vi "rsidr_core_global.vi"() -> ()   [LabVIEW 2015, in "Rohde&Schwarz CMXP GPRF.lvlib"] (continued)
i0, i1, i2, i3, i4, i5, i6, i7, i8, i9, i10, i11, i12, i13, i14, i15, i16, i17, i18, i19, i20, i21, i22, i23, i24, i25, i26, i27, i28, i29, i30, i31, i32\r\n\nRemote-control command(s):\nREAD:GPRF:MEAS<i>:IQRecorder:BIN?"}, {"Level"=3, "Class Only"=FALSE, "Identifier"="RSCMXPGPRF_ATTR_READ_IQ_RECORDER_MEASUREMENT_IQ_AMPLITUDES", "Descriptive Name"="Read IQ Recorder Measurement IQ Amplitudes", "Data Type"=6, "Command"="READ:GPRF:MEAS{instance}:IQR?", "Access"=0, "Range Table"="", "Read Callback"="", "Write Callback"="", "Supported Models"="", "Instrument Options"="", "Flags"=0, "Help"="Returns the I and Q amplitudes in the format specified by FORMat:BASE:DATA.\n\nAvailable Repeated Capabilities:\ninstance: i0, i1, i2, i3, i4, i5, i6, i7, i8, i9, i10, i11, i12, i13, i14, i15, i16, i17, i18, i19, i20, i21, i22, i23, i24, i25, i26, i27, i28, i29, i30, i31, i32\r\n\nRemote-control command(s):\nREAD:GPRF:MEAS<i>:IQRecorder?"}, {"Level"=3, "Class Only"=FALSE, "Identifier"="RSCMXPGPRF_ATTR_FETCH_IQ_RECORDER_MEASUREMENT_IQ_AMPLITUDES", "Descriptive Name"="Fetch IQ Recorder Measurement IQ Amplitudes", "Data Type"=6, "Command"="FETC:GPRF:MEAS{instance}:IQR?", "Access"=0, "Range Table"="", "Read Callback"="", "Write Callback"="", "Supported Models"="", "Instrument Options"="", "Flags"=0, "Help"="Returns the I and Q amplitudes in the format specified by FORMat:BASE:DATA.\n\nAvailable Repeated Capabilities:\ninstance: i0, i1, i2, i3, i4, i5, i6, i7, i8, i9, i10, i11, i12, i13, i14, i15, i16, i17, i18, i19, i20, i21, i22, i23, i24, i25, i26, i27, i28, i29, i30, i31, i32\r\n\nRemote-control command(s):\nFETCh:GPRF:MEAS<i>:IQRecorder?"}, {"Level"=3, "Class Only"=FALSE, "Identifier"="RSCMXPGPRF_ATTR_FETCH_IQ_RECORDER_MEASUREMENT_RELIABILITY", "Descriptive Name"="Fetch IQ Recorder Measurement Reliability", "Data Type"=6, "Command"="FETC:GPRF:MEAS{instance}:IQR:REL?", "Access"=0, "Range Table"="", "Read Callback"="", "Write Callback"="", "Supported Models"="", "Instrument Options"="", "Flags"=0, "Help"="Queries the reliability indicator for the I/Q recorder, see Reliability Indicator.\n\nAvailable Repeated Capabilities:\ninstance: i0, i1, i2, i3, i4, i5, i6, i7, i8, i9, i10, i11, i12, i13, i14, i15, i16, i17, i18, i19, i20, i21, i22, i23, i24, i25, i26, i27, i28, i29, i30, i31, i32\r\n\nRemote-control command(s):\nFETCh:GPRF:MEAS<i>:IQRecorder:RELiability?"}, {"Level"=1, "Class Only"=TRUE, "Identifier"="", "Descriptive Name"="External Power Sensor Measurement", "Data Type"=0, "Command"="", "Access"=0, "Range Table"="", "Read Callback"="", "Write Callback"="", "Supported Models"="", "Instrument Options"="", "Flags"=0, "Help"=""}, {"Level"=2, "Class Only"=TRUE, "Identifier"="", "Descriptive Name"="Configuration", "Data Type"=0, "Command"="", "Access"=0, "Range Table"="", "Read Callback"="", "Write Callback"="", "Supported Models"="", "Instrument Options"="", "Flags"=0, "Help"=""}, {"Level"=3, "Class Only"=FALSE, "Identifier"="RSCMXPGPRF_ATTR_SENSOR_MEASUREMENT_ZEROING", "Descriptive Name"="Sensor Measurement Zeroing", "Data Type"=4, "Command"="CAL:GPRF:MEAS{instance}:EPS:ZERO", "Access"=1, "Range Table"="", "Read Callback"="", "Write Callback"="", "Supported Models"="", "Instrument Options"="", "Flags"=0, "Help"="Initiate zeroing of the power sensor or reads the zeroing state. A running external power sensor measurement is interrupted and re-started after the zeroing procedure has been completed.\n\nAvailable Repeated Capabilities:\ninstance: i0, i1, i2, i3, i4, i5, i6, i7, i8, i9, i10, i11, i12, i13, i14, i15, i16, i17, i18, i19, i20, i21, i22, i23, i24, i25, i26, i27, i28, i29, i30, i31, i32\r\n\nRemote-control command(s):\nCALibration:GPRF:MEAS<i>:EPSensor:ZEROing"}, {"Level"=3, "Class Only"=FALSE, "Identifier"="RSCMXPGPRF_ATTR_QUERY_SENSOR_MEASUREMENT_ZEROING", "Descriptive Name"="Query Sensor Measurement Zeroing", "Data Type"=6, "Command"="CAL:GPRF:MEAS{instance}:EPS:ZERO?", "Access"=0, "Range Table"="", "Read Callback"="", "Write Callback"="", "Supported Models"="", "Instrument Options"="", "Flags"=0, "Help"="Reads status of zeroing of the power sensor.\n\nAvailable Repeated Capabilities:\ninstance: i0, i1, i2, i3, i4, i5, i6, i7, i8, i9, i10, i11, i12, i13, i14, i15, i16, i17, i18, i19, i20, i21, i22, i23, i24, i25, i26, i27, i28, i29, i30, i31, i32\r\n\nRemote-control command(s):\nCALibration:GPRF:MEAS<i>:EPSensor:ZEROing?"}, {"Level"=3, "Class Only"=FALSE, "Identifier"="RSCMXPGPRF_ATTR_SENSOR_MEASUREMENT_REPETITION_MODE", "Descriptive Name"="Sensor Measurement Repetition Mode", "Data Type"=0, "Command"="CONF:GPRF:MEAS{instance}:EPS:REP", "Access"=2, "Range Table"="rsCmxpGprf_rngRepMode", "Read Callback"="", "Write Callback"="", "Supported Models"="", "Instrument Options"="", "Flags"=0, "Help"="Specifies the repetition mode of the measurement; see Statistical Settings. The repetition mode specifies whether the measurement is stopped after a single shot or repeated continuously.\n\nAvailable Repeated Capabilities:\ninstance: i0, i1, i2, i3, i4, i5, i6, i7, i8, i9, i10, i11, i12, i13, i14, i15, i16, i17, i18, i19, i20, i21, i22, i23, i24, i25, i26, i27, i28, i29, i30, i31, i32\r\n\nRemote-control command(s):\nCONFigure:GPRF:MEAS<i>:EPSensor:REPetition"}, {"Level"=3, "Class Only"=FALSE, "Identifier"="RSCMXPGPRF_ATTR_SENSOR_MEASUREMENT_COUNT", "Descriptive Name"="Sensor Measurement Count", "Data Type"=0, "Command"="CONF:GPRF:MEAS{instance}:EPS:SCO", "Access"=2, "Range Table"="rsCmxpGprf_rngStatCount", "Read Callback"="", "Write Callback"="", "Supported Models"="", "Instrument Options"="", "Flags"=0, "Help"="Specifies the statistic count of the measurement; see Statistical Settings. The statistic count is equal to the number of measurement intervals per single shot.\n\nAvailable Repeated Capabilities:\ninstance: i0, i1, i2, i3, i4, i5, i6, i7, i8, i9, i10, i11, i12, i13, i14, i15, i16, i17, i18, i19, i20, i21, i22, i23, i24, i25, i26, i27, i28, i29, i30, i31, i32\r\n\nRemote-control command(s):\nCONFigure:GPRF:MEAS<i>:EPSensor:SCOunt"}, {"Level"=3, "Class Only"=FALSE, "Identifier"="RSCMXPGPRF_ATTR_SENSOR_MEASUREMENT_FREQUENCY", "Descriptive Name"="Sensor Measurement Frequency", "Data Type"=1, "Command"="CONF:GPRF:MEAS{instance}:EPS:FREQ", "Access"=2, "Range Table"="", "Read Callback"="", "Write Callback"="", "Supported Models"="", "Instrument Options"="", "Flags"=0, "Help"="Specifies the input frequency at the power sensor.\n\nAvailable Repeated Capabilities:\ninstance: i0, i1, i2, i3, i4, i5, i6, i7, i8, i9, i10, i11, i12, i13, i14, i15, i16, i17, i18, i19, i20, i21, i22, i23, i24, i25, i26, i27, i28, i29, i30, i31, i32\r\n\nRemote-control command(s):\nCONFigure:GPRF:MEAS<i>:EPSensor:FREQuency"}, {"Level"=3, "Class Only"=FALSE, "Identifier"="RSCMXPGPRF_ATTR_SENSOR_MEASUREMENT_ATTENUATION_STATE", "Descriptive Name"="Sensor Measurement Attenuation State", "Data Type"=3, "Command"="CONF:GPRF:MEAS{instance}:EPS:ATT:STAT", "Access"=2, "Range Table"="", "Read Callback"="", "Write Callback"="", "Supported Models"="", "Instrument Options"="", "Flags"=0, "Help"="Enables or disables an external input attenuation at the sensor.\n\nAvailable Repeated Capabilities:\ninstance: i0, i1, i2, i3, i4, i5, i6, i7, i8, i9, i10, i11, i12, i13, i14, i15, i16, i17, i18, i19, i20, i21, i22, i23, i24, i25, i26, i27, i28, i29, i30, i31, i32\r\n\nRemote-control command(s):\nCONFigure:GPRF:MEAS<i>:EPSensor:ATTenuation:STATe"}, {"Level"=3, "Class Only"=FALSE, "Identifier"="RSCMXPGPRF_ATTR_SENSOR_MEASUREMENT_ATTENUATION", "Descriptive Name"="Sensor Measurement Attenuation", "Data Type"=1, "Command"="CONF:GPRF:MEAS{instance}:EPS:ATT", "Access"=2, "Range Table"="rsCmxpGprf_rngExtSensorAttenuation", "Read Callback"="", "Write Callback"="", "Supported Models"="", "Instrument Options"="", "Flags"=0, "Help"="Specifies the external input attenuation factor to correct the power reading at the sensor.\n\nAvailable Repeated Capabilities:\ninstance: i0, i1, i2, i3, i4, i5, i6, i7, i8, i9, i10, i11, i12, i13, i14, i15, i16, i17, i18, i19, i20, i21, i22, i23, i24, i25, i26, i27, i28, i29, i30, i31, i32\r\n\nRemote-control command(s):\nCONFigure:GPRF:MEAS<i>:EPSensor:ATTenuation"}, {"Level"=3, "Class Only"=FALSE, "Identifier"="RSCMXPGPRF_ATTR_SENSOR_MEASUREMENT_RESOLUTION", "Descriptive Name"="Sensor Measurement Resolution", "Data Type"=0, "Command"="CONF:GPRF:MEAS{instance}:EPS:RES", "Access"=2, "Range Table"="rsCmxpGprf_rngResolution", "Read Callback"="", "Write Callback"="", "Supported Models"="", "Instrument Options"="", "Flags"=0, "Help"="Defines the number of digits of the power results in the measurement dialog. This command does not affect the remote control results.\n\nAvailable Repeated Capabilities:\ninstance: i0, i1, i2, i3, i4, i5, i6, i7, i8, i9, i10, i11, i12, i13, i14, i15, i16, i17, i18, i19, i20, i21, i22, i23, i24, i25, i26, i27, i28, i29, i30, i31, i32\r\n\nRemote-control command(s):\nCONFigure:GPRF:MEAS<i>:EPSensor:RESolution"}, {"Level"=3, "Class Only"=FALSE, "Identifier"="RSCMXPGPRF_ATTR_POWER_SENSOR_MEASUREMENT_TIMEOUT", "Descriptive Name"="Power Sensor Measurement Timeout", "Data Type"=1, "Command"="CONF:GPRF:MEAS{instance}:EPS:TOUT", "Access"=2, "Range Table"="", "Read Callback"="", "Write Callback"="", "Supported Models"="", "Instrument Options"="", "Flags"=0, "Help"="Defines a timeout for the measurement.\n\nAvailable Repeated Capabilities:\ninstance: i0, i1, i2, i3, i4, i5, i6, i7, i8, i9, i10, i11, i12, i13, i14, i15, i16, i17, i18, i19, i20, i21, i22, i23, i24, i25, i26, i27, i28, i29, i30, i31, i32\r\n\nRemote-control command(s):\nCONFigure:GPRF:MEAS<i>:EPSensor:TOUT"}, {"Level"=2, "Class Only"=TRUE, "Identifier"="", "Descriptive Name"="Control", "Data Type"=0, "Command"="", "Access"=0, "Range Table"="", "Read Callback"="", "Write Callback"="", "Supported Models"="", "Instrument Options"="", "Flags"=0, "Help"=""}, {"Level"=3, "Class Only"=FALSE, "Identifier"="RSCMXPGPRF_ATTR_SENSOR_MEASUREMENT_INIT", "Descriptive Name"="Sensor Measurement Init", "Data Type"=4, "Command"="INIT:GPRF:MEAS{instance}:EPS", "Access"=1, "Range Table"="", "Read Callback"="", "Write Callback"="", "Supported Models"="", "Instrument Options"="", "Flags"=0, "Help"="Starts or restarts the measurement; the R&S CMW 500 enters the &apos;RUN&apos; state.\n\nAvailable Repeated Capabilities:\ninstance: i0, i1, i2, i3, i4, i5, i6, i7, i8, i9, i10, i11, i12, i13, i14, i15, i16, i17, i18, i19, i20, i21, i22, i23, i24, i25, i26, i27, i28, i29, i30, i31, i32\r\n\nRemote-control command(s):\nINITiate:GPRF:MEAS<i>:EPSensor"}, {"Level"=3, "Class Only"=FALSE, "Identifier"="RSCMXPGPRF_ATTR_SENSOR_MEASUREMENT_ABORT", "Descriptive Name"="Sensor Measurement Abort", "Data Type"=4, "Command"="ABOR:GPRF:MEAS{instance}:EPS", "Access"=1, "Range Table"="", "Read Callback"="", "Write Callback"="", "Supported Models"="", "Instrument Options"="", "Flags"=0, "Help"="Causes a running measurement to stop immediately; the R&S CMW 500 enters the &apos;OFF&apos; state.\n\nAvailable Repeated Capabilities:\ninstance: i0, i1, i2, i3, i4, i5, i6, i7, i8, i9, i10, i11, i12, i13, i14, i15, i16, i17, i18, i19, i20, i21, i22, i23, i24, i25, i26, i27, i28, i29, i30, i31, i32\r\n\nRemote-control command(s):\nABORt:GPRF:MEAS<i>:EPSensor"}, {"Level"=3, "Class Only"=FALSE, "Identifier"="RSCMXPGPRF_ATTR_SENSOR_MEASUREMENT_STOP", "Descriptive Name"="Sensor Measurement Stop", "Data Type"=4, "Command"="STOP:GPRF:MEAS{instance}:EPS", "Access"=1, "Range Table"="", "Read Callback"="", "Write Callback"="", "Supported Models"="", "Instrument Options"="", "Flags"=0, "Help"="Causes a running measurement to stop after the current evaluation period is terminated and valid results are available; the R&S CMW 500 enters the &apos;RDY&apos; state.\n\nAvailable Repeated Capabilities:\ninstance: i0, i1, i2, i3, i4, i5, i6, i7, i8, i9, i10, i11, i12, i13, i14, i15, i16, i17, i18, i19, i20, i21, i22, i23, i24, i25, i26, i27, i28, i29, i30, i31, i32\r\n\nRemote-control command(s):\nSTOP:GPRF:MEAS<i>:EPSensor"}, {"Level"=3, "Class Only"=FALSE, "Identifier"="RSCMXPGPRF_ATTR_SENSOR_MEASUREMENT_IDN", "Descriptive Name"="Sensor Measurement IDN", "Data Type"=2, "Command"="FETC:GPRF:MEAS{instance}:EPS:IDN?", "Access"=0, "Range Table"="", "Read Callback"="", "Write Callback"="", "Supported Models"="", "Instrument Options"="", "Flags"=0, "Help"="Returns the identification string of the connected external sensor.\n\nAvailable Repeated Capabilities:\ninstance: i0, i1, i2, i3, i4, i5, i6, i7, i8, i9, i10, i11, i12, i13, i14, i15, i16, i17, i18, i19, i20, i21, i22, i23, i24, i25, i26, i27, i28, i29, i30, i31, i32\r\n\nRemote-control command(s):\nFETCh:GPRF:MEAS<i>:EPSensor:IDN?"}, {"Level"=3, "Class Only"=FALSE, "Identifier"="RSCMXPGPRF_ATTR_SENSOR_MEASUREMENT_STATUS", "Descriptive Name"="Sensor Measurement Status", "Data Type"=6, "Command"="FETC:GPRF:MEAS{instance}:EPS:STAT?", "Access"=0, "Range Table"="", "Read Callback"="", "Write Callback"="", "Supported Models"="", "Instrument Options"="", "Flags"=0, "Help"="Queries the main measurement state.\n\nAvailable Repeated Capabilities:\ninstance: i0, i1, i2, i3, i4, i5, i6, i7, i8, i9, i10, i11, i12, i13, i14, i15, i16, i17, i18, i19, i20, i21, i22, i23, i24, i25, i26, i27, i28, i29, i30, i31, i32\r\n\nRemote-control command(s):\nFETCh:GPRF:MEAS<i>:EPSensor:STATe?"}, {"Level"=3, "Class Only"=FALSE, "Identifier"="RSCMXPGPRF_ATTR_SENSOR_MEASUREMENT_STATUS_ALL", "Descriptive Name"="Sensor Measurement Status All", "Data Type"=6, "Command"="FETC:GPRF:MEAS{instance}:EPS:STAT:ALL?", "Access"=0, "Range Table"="", "Read Callback"="", "Write Callback"="", "Supported Models"="", "Instrument Options"="", "Flags"=0, "Help"="Queries the main measurement state and the measurement substates. Both measurement substates are relevant for running measurements only. Use FETCh:...:STATe? to query the main measurement state only. Use INITiate..., STOP..., ABORt... to change the measurement state.\n\nAvailable Repeated Capabilities:\ninstance: i0, i1, i2, i3, i4, i5, i6, i7, i8, i9, i10, i11, i12, i13, i14, i15, i16, i17, i18, i19, i20, i21, i22, i23, i24, i25, i26, i27, i28, i29, i30, i31, i32\r\n\nRemote-control command(s):\nFETCh:GPRF:MEAS<i>:EPSensor:STATe:ALL?"}, {"Level"=2, "Class Only"=TRUE, "Identifier"="", "Descriptive Name"="Results", "Data Type"=0, "Command"="", "Access"=0, "Range Table"="", "Read Callback"="", "Write Callback"="", "Supported Models"="", "Instrument Options"="", "Flags"=0, "Help"="Contains attributes for Power Sensor Results."}, {"Level"=3, "Class Only"=FALSE, "Identifier"="RSCMXPGPRF_ATTR_READ_POWER_SENSOR", "Descriptive Name"="Read Power Sensor", "Data Type"=6, "Command"="READ:GPRF:MEAS{instance}:EPS?", "Access"=0, "Range Table"="", "Read Callback"="", "Write Callback"="", "Supported Models"="", "Instrument Options"="", "Flags"=0, "Help"="Returns all results of the EPS measurement.\n\nAvailable Repeated Capabilities:\ninstance: i0, i1, i2, i3, i4, i5, i6, i7, i8, i9, i10, i11, i12, i13, i14, i15, i16, i17, i18, i19, i20, i21, i22, i23, i24, i25, i26, i27, i28, i29, i30, i31, i32\r\n\nRemote-control command(s):\nREAD:GPRF:MEAS<i>:EPSensor?"}, {"Level"=3, "Class Only"=FALSE, "Identifier"="RSCMXPGPRF_ATTR_FETCH_POWER_SENSOR", "Descriptive Name"="Fetch Power Sensor", "Data Type"=6, "Command"="FETC:GPRF:MEAS{instance}:EPS?", "Access"=0, "Range Table"="", "Read Callback"="", "Write Callback"="", "Supported Models"="", "Instrument Options"="", "Flags"=0, "Help"="Returns all results of the EPS measurement.\n\nAvailable Repeated Capabilities:\ninstance: i0, i1, i2, i3, i4, i5, i6, i7, i8, i9, i10, i11, i12, i13, i14, i15, i16, i17, i18, i19, i20, i21, i22, i23, i24, i25, i26, i27, i28, i29, i30, i31, i32\r\n\nRemote-control command(s):\nFETCh:GPRF:MEAS<i>:EPSensor?"}, {"Level"=1, "Class Only"=TRUE, "Identifier"="", "Descriptive Name"="FFT Spectrum Analyzer", "Data Type"=0, "Command"="", "Access"=0, "Range Table"="", "Read Callback"="", "Write Callback"="", "Supported Models"="", "Instrument Options"="", "Flags"=0, "Help"=""}, {"Level"=2, "Class Only"=TRUE, "Identifier"="", "Descriptive Name"="Configuration", "Data Type"=0, "Command"="", "Access"=0, "Range Table"="", "Read Callback"="", "Write Callback"="", "Supported Models"="", "Instrument Options"="", "Flags"=0, "Help"=""}, {"Level"=3, "Class Only"=FALSE, "Identifier"="RSCMXPGPRF_ATTR_FFT_MEASUREMENT_REPETITION_MODE", "Descriptive Name"="FFT Measurement Repetition Mode", "Data Type"=0, "Command"="CONF:GPRF:MEAS{instance}:FFTS:REP", "Access"=2, "Range Table"="rsCmxpGprf_rngRepMode", "Read Callback"="", "Write Callback"="", "Supported Models"="", "Instrument Options"="", "Flags"=0, "Help"="Specifies the repetition mode of the measurement; see Statistical Settings. The repetition mode specifies whether the measurement is stopped after a single shot or repeated continuously.\n\nAvailable Repeated Capabilities:\ninstance: i0, i1, i2, i3, i4, i5, i6, i7, i8, i9, i10, i11, i12, i13, i14, i15, i16, i17, i18, i19, i20, i21, i22, i23, i24, i25, i26, i27, i28, i29, i30, i31, i32\r\n\nRemote-control command(s):\nCONFigure:GPRF:MEAS<i>:FFTSanalyzer:REPetition"}, {"Level"=3, "Class Only"=FALSE, "Identifier"="RSCMXPGPRF_ATTR_FFT_MEASUREMENT_TIMEOUT", "Descriptive Name"="FFT Measurement Timeout", "Data Type"=1, "Command"="CONF:GPRF:MEAS{instance}:FFTS:TOUT", "Access"=2, "Range Table"="", "Read Callback"="", "Write Callback"="", "Supported Models"="", "Instrument Options"="", "Flags"=0, "Help"="Defines a timeout for the measurement.\n\nAvailable Repeated Capabilities:\ninstance: i0, i1, i2, i3, i4, i5, i6, i7, i8, i9, i10, i11, i12, i13, i14, i15, i16, i17, i18, i19, i20, i21, i22, i23, i24, i25, i26, i27, i28, i29, i30, i31, i32\r\n\nRemote-control command(s):\nCONFigure:GPRF:MEAS<i>:FFTSanalyzer:TOUT"}, {"Level"=3, "Class Only"=FALSE, "Identifier"="RSCMXPGPRF_ATTR_FFT_MEASUREMENT_COUNT", "Descriptive Name"="FFT Measurement Count", "Data Type"=0, "Command"="CONF:GPRF:MEAS{instance}:FFTS:SCO", "Access"=2, "Range Table"="rsCmxpGprf_rngStatCount", "Read Callback"="", "Write Callback"="", "Supported Models"="", "Instrument Options"="", "Flags"=0, "Help"="Specifies the statistic count of the measurement; see Statistical Settings. The statistic count is equal to the number of measurement intervals per single shot.\n\nAvailable Repeated Capabilities:\ninstance: i0, i1, i2, i3, i4, i5, i6, i7, i8, i9, i10, i11, i12, i13, i14, i15, i16, i17, i18, i19, i20, i21, i22, i23, i24, i25, i26, i27, i28, i29, i30, i31, i32\r\n\nRemote-control command(s):\nCONFigure:GPRF:MEAS<i>:FFTSanalyzer:SCOunt"}, {"Level"=3, "Class Only"=FALSE, "Identifier"="RSCMXPGPRF_ATTR_FFT_MEASUREMENT_RESULTS_REJECTION", "Descriptive Name"="FFT Measurement Results Rejection", "Data Type"=3, "Command"="CONF:GPRF:MEAS{instance}:FFTS:MOEX", "Access"=2, "Range Table"="", "Read Callback"="", "Write Callback"="", "Supported Models"="", "Instrument Options"="", "Flags"=0, "Help"="Specifies whether measurement results that the R&S CMW identifies as faulty or inaccurate are rejected.\n\nAvailable Repeated Capabilities:\ninstance: i0, i1, i2, i3, i4, i5, i6, i7, i8, i9, i10, i11, i12, i13, i14, i15, i16, i17, i18, i19, i20, i21, i22, i23, i24, i25, i26, i27, i28, i29, i30, i31, i32\r\n\nRemote-control command(s):\nCONFigure:GPRF:MEAS<i>:FFTSanalyzer:MOEXception"}, {"Level"=3, "Class Only"=FALSE, "Identifier"="RSCMXPGPRF_ATTR_FFT_MEASUREMENT_FREQUENCY_SPAN", "Descriptive Name"="FFT Measurement Frequency Span", "Data Type"=1, "Command"="CONF:GPRF:MEAS{instance}:FFTS:FSP", "Access"=2, "Range Table"="rsCmxpGprf_rngFFTFrequencySpan", "Read Callback"="", "Write Callback"="", "Supported Models"="", "Instrument Options"="", "Flags"=0, "Help"="Selects the calculated and displayed frequency range (span) of the FFT spectrum analyzer.\n\nAvailable Repeated Capabilities:\ninstance: i0, i1, i2, i3, i4, i5, i6, i7, i8, i9, i10, i11, i12, i13, i14, i15, i16, i17, i18, i19, i20, i21, i22, i23, i24, i25, i26, i27, i28, i29, i30, i31, i32\r\n\nRemote-control command(s):\nCONFigure:GPRF:MEAS<i>:FFTSanalyzer:FSPan"}, {"Level"=3, "Class Only"=FALSE, "Identifier"="RSCMXPGPRF_ATTR_FFT_MEASUREMENT_FFT_LENGTH", "Descriptive Name"="FFT Measurement FFT Length", "Data Type"=0, "Command"="CONF:GPRF:MEAS{instance}:FFTS:FFTL", "Access"=2, "Range Table"="rsCmxpGprf_rngFFTLength", "Read Callback"="", "Write Callback"="", "Supported Models"="", "Instrument Options"="", "Flags"=0, "Help"="Selects the number of samples (FFT Length) that the R&S CMW uses for the FFT analysis.\n\nAvailable Repeated Capabilities:\ninstance: i0, i1, i2, i3, i4, i5, i6, i7, i8, i9, i10, i11, i12, i13, i14, i15, i16, i17, i18, i19, i20, i21, i22, i23, i24, i25, i26, i27, i28, i29, i30, i31, i32\r\n\nRemote-control command(s):\nCONFigure:GPRF:MEAS<i>:FFTSanalyzer:FFTLength"}, {"Level"=3, "Class Only"=FALSE, "Identifier"="RSCMXPGPRF_ATTR_FFT_MEASUREMENT_DETECTOR", "Descriptive Name"="FFT Measurement Detector", "Data Type"=0, "Command"="CONF:GPRF:MEAS{instance}:FFTS:DET", "Access"=2, "Range Table"="rsCmxpGprf_rngFFTDetector", "Read Callback"="", "Write Callback"="", "Supported Models"="", "Instrument Options"="", "Flags"=0, "Help"="Selects the detector for the display of the FFT trace.\n\nAvailable Repeated Capabilities:\ninstance: i0, i1, i2, i3, i4, i5, i6, i7, i8, i9, i10, i11, i12, i13, i14, i15, i16, i17, i18, i19, i20, i21, i22, i23, i24, i25, i26, i27, i28, i29, i30, i31, i32\r\n\nRemote-control command(s):\nCONFigure:GPRF:MEAS<i>:FFTSanalyzer:DETector"}, {"Level"=3, "Class Only"=FALSE, "Identifier"="RSCMXPGPRF_ATTR_FFT_MEASUREMENT_AVERAGING_MODE", "Descriptive Name"="FFT Measurement Averaging Mode", "Data Type"=0, "Command"="CONF:GPRF:MEAS{instance}:FFTS:AMOD", "Access"=2, "Range Table"="rsCmxpGprf_rngLinLog", "Read Callback"="", "Write Callback"="", "Supported Models"="", "Instrument Options"="", "Flags"=0, "Help"="Selects the averaging mode for the average FFT trace.\n\nAvailable Repeated Capabilities:\ninstance: i0, i1, i2, i3, i4, i5, i6, i7, i8, i9, i10, i11, i12, i13, i14, i15, i16, i17, i18, i19, i20, i21, i22, i23, i24, i25, i26, i27, i28, i29, i30, i31, i32\r\n\nRemote-control command(s):\nCONFigure:GPRF:MEAS<i>:FFTSanalyzer:AMODe"}, {"Level"=3, "Class Only"=FALSE, "Identifier"="RSCMXPGPRF_ATTR_FFT_MEASUREMENT_TRIGGER_SOURCE", "Descriptive Name"="FFT Measurement Trigger Source", "Data Type"=2, "Command"="TRIG:GPRF:MEAS{instance}:FFTS:SOUR", "Access"=2, "Range Table"="", "Read Callback"="", "Write Callback"="", "Supported Models"="", "Instrument Options"="", "Flags"=0, "Help"="Selects the source of the trigger events.\n\nAvailable Repeated Capabilities:\ninstance: i0, i1, i2, i3, i4, i5, i6, i7, i8, i9, i10, i11, i12, i13, i14, i15, i16, i17, i18, i19, i20, i21, i22, i23, i24, i25, i26, i27, i28, i29, i30, i31, i32\r\n\nRemote-control command(s):\nTRIGger:GPRF:MEAS<i>:FFTSanalyzer:SOURce"}, {"Level"=3, "Class Only"=FALSE, "Identifier"="RSCMXPGPRF_ATTR_FFT_MEASUREMENT_TRIGGER_SLOPE", "Descriptive Name"="FFT Measurement Trigger Slope", "Data Type"=0, "Command"="TRIG:GPRF:MEAS{instance}:FFTS:SLOP", "Access"=2, "Range Table"="rsCmxpGprf_rngTrigSlope", "Read Callback"="", "Write Callback"="", "Supported Models"="", "Instrument Options"="", "Flags"=0, "Help"="Qualifies whether the trigger event is generated at the rising or at the falling edge of the trigger pulse (valid for the power trigger sources.\n\nAvailable Repeated Capabilities:\ninstance: i0, i1, i2, i3, i4, i5, i6, i7, i8, i9, i10, i11, i12, i13, i14, i15, i16, i17, i18, i19, i20, i21, i22, i23, i24, i25, i26, i27, i28, i29, i30, i31, i32\r\n\nRemote-control command(s):\nTRIGger:GPRF:MEAS<i>:FFTSanalyzer:SLOPe"}, {"Level"=3, "Class Only"=FALSE, "Identifier"="RSCMXPGPRF_ATTR_FFT_MEASUREMENT_TRIGGER_THRESHOLD", "Descriptive Name"="FFT Measurement Trigger Threshold", "Data Type"=1, "Command"="TRIG:GPRF:MEAS{instance}:FFTS:THR", "Access"=2, "Range Table"="rsCmxpGprf_rngTrigThreshold", "Read Callback"="", "Write Callback"="", "Supported Models"="", "Instrument Options"="", "Flags"=0, "Help"="Defines the trigger threshold for the power trigger sources.\n\nAvailable Repeated Capabilities:\ninstance: i0, i1, i2, i3, i4, i5, i6, i7, i8, i9, i10, i11, i12, i13, i14, i15, i16, i17, i18, i19, i20, i21, i22, i23, i24, i25, i26, i27, i28, i29, i30, i31, i32\r\n\nRemote-control command(s):\nTRIGger:GPRF:MEAS<i>:FFTSanalyzer:THReshold"}, {"Level"=3, "Class Only"=FALSE, "Identifier"="RSCMXPGPRF_ATTR_FFT_MEASUREMENT_TRIGGER_OFFSET", "Descriptive Name"="FFT Measurement Trigger Offset", "Data Type"=1, "Command"="TRIG:GPRF:MEAS{instance}:FFTS:OFFS", "Access"=2, "Range Table"="rsCmxpGprf_rngTrigOffset", "Read Callback"="", "Write Callback"="", "Supported Models"="", "Instrument Options"="", "Flags"=0, "Help"="Defines a delay time for the Internal Trigger (Internal). The trigger offset delays the start of the measurement relative to the trigger event.\n\nAvailable Repeated Capabilities:\ninstance: i0, i1, i2, i3, i4, i5, i6, i7, i8, i9, i10, i11, i12, i13, i14, i15, i16, i17, i18, i19, i20, i21, i22, i23, i24, i25, i26, i27, i28, i29, i30, i31, i32\r\n\nRemote-control command(s):\nTRIGger:GPRF:MEAS<i>:FFTSanalyzer:OFFSet"}, {"Level"=3, "Class Only"=FALSE, "Identifier"="RSCMXPGPRF_ATTR_FFT_MEASUREMENT_TRIGGER_OFFSET_MODE", "Descriptive Name"="FFT Measurement Trigger Offset Mode", "Data Type"=0, "Command"="TRIG:GPRF:MEAS{instance}:FFTS:OMOD", "Access"=2, "Range Table"="rsCmxpGprf_rngFFTTriggerOffsetMode", "Read Callback"="", "Write Callback"="", "Supported Models"="", "Instrument Options"="", "Flags"=0, "Help"="Selects a fixed or a variable trigger offset. In the &apos;FFT Spectrum Analyzer&apos; measurement, the trigger offset defines the center of the FFT window.\n\nAvailable Repeated Capabilities:\ninstance: i0, i1, i2, i3, i4, i5, i6, i7, i8, i9, i10, i11, i12, i13, i14, i15, i16, i17, i18, i19, i20, i21, i22, i23, i24, i25, i26, i27, i28, i29, i30, i31, i32\r\n\nRemote-control command(s):\nTRIGger:GPRF:MEAS<i>:FFTSanalyzer:OMODe"}, {"Level"=3, "Class Only"=FALSE, "Identifier"="RSCMXPGPRF_ATTR_FFT_MEASUREMENT_TRIGGER_TIMEOUT", "Descriptive Name"="FFT Measurement Trigger Timeout", "Data Type"=1, "Command"="TRIG:GPRF:MEAS{instance}:FFTS:TOUT", "Access"=2, "Range Table"="rsCmxpGprf_rngTrigTout", "Read Callback"="", "Write Callback"="", "Supported Models"="", "Instrument Options"="", "Flags"=0, "Help"="Sets a time after which the initiated measurement is automatically terminated if it does not receive a trigger event.\n\nAvailable Repeated Capabilities:\ninstance: i0, i1, i2, i3, i4, i5, i6, i7, i8, i9, i10, i11, i12, i13, i14, i15, i16, i17, i18, i19, i20, i21, i22, i23, i24, i25, i26, i27, i28, i29, i30, i31, i32\r\n\nRemote-control command(s):\nTRIGger:GPRF:MEAS<i>:FFTSanalyzer:TOUT"}, {"Level"=3, "Class Only"=FALSE, "Identifier"="RSCMXPGPRF_ATTR_FFT_MEASUREMENT_TRIGGER_TIMEOUT_ENABLED", "Descriptive Name"="FFT Measurement Trigger Timeout Enabled", "Data Type"=3, "Command"="TRIG:GPRF:MEAS{instance}:FFTS:TOUT", "Access"=2, "Range Table"="", "Read Callback"="", "Write Callback"="", "Supported Models"="", "Instrument Options"="", "Flags"=0, "Help"="Disables timeout | enables timeout using the previous/default values.\n\nAvailable Repeated Capabilities:\ninstance: i0, i1, i2, i3, i4, i5, i6, i7, i8, i9, i10, i11, i12, i13, i14, i15, i16, i17, i18, i19, i20, i21, i22, i23, i24, i25, i26, i27, i28, i29, i30, i31, i32\r\n\nRemote-control command(s):\nTRIGger:GPRF:MEAS<i>:FFTSanalyzer:TOUT"}, {"Level"=3, "Class Only"=FALSE, "Identifier"="RSCMXPGPRF_ATTR_FFT_MEASUREMENT_TRIGGER_GAP", "Descriptive Name"="FFT Measurement Trigger Gap", "Data Type"=1, "Command"="TRIG:GPRF:MEAS{instance}:FFTS:MGAP", "Access"=2, "Range Table"="rsCmxpGprf_rngTriggerGap", "Read Callback"="", "Write Callback"="", "Supported Models"="", "Instrument Options"="", "Flags"=0, "Help"="Defines a minimum duration of the power-down periods (gaps) between two triggered IF power pulses.\n\nAvailable Repeated Capabilities:\ninstance: i0, i1, i2, i3, i4, i5, i6, i7, i8, i9, i10, i11, i12, i13, i14, i15, i16, i17, i18, i19, i20, i21, i22, i23, i24, i25, i26, i27, i28, i29, i30, i31, i32\r\n\nRemote-control command(s):\nTRIGger:GPRF:MEAS<i>:FFTSanalyzer:MGAP"}, {"Level"=3, "Class Only"=FALSE, "Identifier"="RSCMXPGPRF_ATTR_FFT_MEASUREMENT_PEAK_SEARCH_MARKERS", "Descriptive Name"="FFT Measurement Peak Search Markers", "Data Type"=0, "Command"="CONF:GPRF:MEAS{instance}:FFTS:PSE:NOAM", "Access"=2, "Range Table"="rsCmxpGprf_rngPeakSearchMarkers", "Read Callback"="", "Write Callback"="", "Supported Models"="", "Instrument Options"="", "Flags"=0, "Help"="Defines the number of active markers for the peak search.\n\nAvailable Repeated Capabilities:\ninstance: i0, i1, i2, i3, i4, i5, i6, i7, i8, i9, i10, i11, i12, i13, i14, i15, i16, i17, i18, i19, i20, i21, i22, i23, i24, i25, i26, i27, i28, i29, i30, i31, i32\r\n\nRemote-control command(s):\nCONFigure:GPRF:MEAS<i>:FFTSanalyzer:PSEarch:NOAMarkers"}, {"Level"=3, "Class Only"=FALSE, "Identifier"="RSCMXPGPRF_ATTR_FFT_MEASUREMENT_TRIGGER_SOURCE_CATALOG", "Descriptive Name"="FFT Measurement Trigger Source Catalog", "Data Type"=2, "Command"="TRIG:GPRF:MEAS{instance}:FFTS:CAT:SOUR?", "Access"=0, "Range Table"="", "Read Callback"="", "Write Callback"="", "Supported Models"="", "Instrument Options"="", "Flags"=0, "Help"="Lists all trigger source values that can be set using TRIGger:GPRF:MEAS<i>:FFTSanalyzer:SOURce.\n\nAvailable Repeated Capabilities:\ninstance: i0, i1, i2, i3, i4, i5, i6, i7, i8, i9, i10, i11, i12, i13, i14, i15, i16, i17, i18, i19, i20, i21, i22, i23, i24, i25, i26, i27, i28, i29, i30, i31, i32\r\n\nRemote-control command(s):\nTRIGger:GPRF:MEAS<i>:FFTSanalyzer:CATalog:SOURce?"}, {"Level"=3, "Class Only"=FALSE, "Identifier"="RSCMXPGPRF_ATTR_FFT_MEASUREMENT_PEAK_SEARCH", "Descriptive Name"="FFT Measurement Peak Search", "Data Type"=6, "Command"="CONF:GPRF:MEAS{instance}:FFTS:PSE", "Access"=2, "Range Table"="", "Read Callback"="", "Write Callback"="", "Supported Models"="", "Instrument Options"="", "Flags"=0, "Help"="Defines the peak search ranges. The maximum allowed search ranges depend on the frequency span: span/2 to span/2.\n\nAvailable Repeated Capabilities:\ninstance: i0, i1, i2, i3, i4, i5, i6, i7, i8, i9, i10, i11, i12, i13, i14, i15, i16, i17, i18, i19, i20, i21, i22, i23, i24, i25, i26, i27, i28, i29, i30, i31, i32\r\n\nRemote-control command(s):\nCONFigure:GPRF:MEAS<i>:FFTSanalyzer:PSEarch"}, {"Level"=2, "Class Only"=TRUE, "Identifier"="", "Descriptive Name"="Control", "Data Type"=0, "Command"="", "Access"=0, "Range Table"="", "Read Callback"="", "Write Callback"="", "Supported Models"="", "Instrument Options"="", "Flags"=0, "Help"=""}, {"Level"=3, "Class Only"=FALSE, "Identifier"="RSCMXPGPRF_ATTR_FFT_MEASUREMENT_INIT", "Descriptive Name"="FFT Measurement Init", "Data Type"=4, "Command"="INIT:GPRF:MEAS{instance}:FFTS", "Access"=1, "Range Table"="", "Read Callback"="", "Write Callback"="", "Supported Models"="", "Instrument Options"="", "Flags"=0, "Help"="Starts or restarts the measurement; the R&S CMW 500 enters the &apos;RUN&apos; state.\n\nAvailable Repeated Capabilities:\ninstance: i0, i1, i2, i3, i4, i5, i6, i7, i8, i9, i10, i11, i12, i13, i14, i15, i16, i17, i18, i19, i20, i21, i22, i23, i24, i25, i26, i27, i28, i29, i30, i31, i32\r\n\nRemote-control command(s):\nINITiate:GPRF:MEAS<i>:FFTSanalyzer"}, {"Level"=3, "Class Only"=FALSE, "Identifier"="RSCMXPGPRF_ATTR_FFT_MEASUREMENT_ABORT", "Descriptive Name"="FFT Measurement Abort", "Data Type"=4, "Command"="ABOR:GPRF:MEAS{instance}:FFTS", "Access"=1, "Range Table"="", "Read Callback"="", "Write Callback"="", "Supported Models"="", "Instrument Options"="", "Flags"=0, "Help"="Causes a running measurement to stop immediately; the R&S CMW 500 enters the &apos;OFF&apos; state.\n\nAvailable Repeated Capabilities:\ninstance: i0, i1, i2, i3, i4, i5, i6, i7, i8, i9, i10, i11, i12, i13, i14, i15, i16, i17, i18, i19, i20, i21, i22, i23, i24, i25, i26, i27, i28, i29, i30, i31, i32\r\n\nRemote-control command(s):\nABORt:GPRF:MEAS<i>:FFTSanalyzer"}, {"Level"=3, "Class Only"=FALSE, "Identifier"="RSCMXPGPRF_ATTR_FFT_MEASUREMENT_STOP", "Descriptive Name"="FFT Measurement Stop", "Data Type"=4, "Command"="STOP:GPRF:MEAS{instance}:FFTS", "Access"=1, "Range Table"="", "Read Callback"="", "Write Callback"="", "Supported Models"="", "Instrument Options"="", "Flags"=0, "Help"="Causes a running measurement to stop after the current evaluation period is terminated and valid results are available; the R&S CMW 500 enters the &apos;RDY&apos; state.\n\nAvailable Repeated Capabilities:\ninstance: i0, i1, i2, i3, i4, i5, i6, i7, i8, i9, i10, i11, i12, i13, i14, i15, i16, i17, i18, i19, i20, i21, i22, i23, i24, i25, i26, i27, i28, i29, i30, i31, i32\r\n\nRemote-control command(s):\nSTOP:GPRF:MEAS<i>:FFTSanalyzer"}, {"Level"=3, "Class Only"=FALSE, "Identifier"="RSCMXPGPRF_ATTR_FFT_MEASUREMENT_STATUS", "Descriptive Name"="FFT Measurement Status", "Data Type"=6, "Command"="FETC:GPRF:MEAS{instance}:FFTS:STAT?", "Access"=0, "Range Table"="", "Read Callback"="", "Write Callback"="", "Supported Models"="", "Instrument Options"="", "Flags"=0, "Help"="Queries the main measurement state.\n\nAvailable Repeated Capabilities:\ninstance: i0, i1, i2, i3, i4, i5, i6, i7, i8, i9, i10, i11, i12, i13, i14, i15, i16, i17, i18, i19, i20, i21, i22, i23, i24, i25, i26, i27, i28, i29, i30, i31, i32\r\n\nRemote-control command(s):\nFETCh:GPRF:MEAS<i>:FFTSanalyzer:STATe?"}, {"Level"=3, "Class Only"=FALSE, "Identifier"="RSCMXPGPRF_ATTR_FFT_MEASUREMENT_STATUS_ALL", "Descriptive Name"="FFT Measurement Status All", "Data Type"=6, "Command"="FETC:GPRF:MEAS{instance}:FFTS:STAT:ALL?", "Access"=0, "Range Table"="", "Read Callback"="", "Write Callback"="", "Supported Models"="", "Instrument Options"="", "Flags"=0, "Help"="Queries the main measurement state and the measurement substates. Both measurement substates are relevant for running measurements only. Use FETCh:...:STATe? to query the main measurement state only. Use INITiate..., STOP..., ABORt... to change the measurement state.\n\nAvailable Repeated Capabilities:\ninstance: i0, i1, i2, i3, i4, i5, i6, i7, i8, i9, i10, i11, i12, i13, i14, i15, i16, i17, i18, i19, i20, i21, i22, i23, i24, i25, i26, i27, i28, i29, i30, i31, i32\r\n\nRemote-control command(s):\nFETCh:GPRF:MEAS<i>:FFTSanalyzer:STATe:ALL?"}, {"Level"=2, "Class Only"=TRUE, "Identifier"="", "Descriptive Name"="Results", "Data Type"=0, "Command"="", "Access"=0, "Range Table"="", "Read Callback"="", "Write Callback"="", "Supported Models"="", "Instrument Options"="", "Flags"=0, "Help"="Contains attributes for FFT Measurement Results."}, {"Level"=3, "Class Only"=FALSE, "Identifier"="RSCMXPGPRF_ATTR_READ_FFT_MEASUREMENT_POWER_CURRENT", "Descriptive Name"="Read FFT Measurement Power Current", "Data Type"=6, "Command"="READ:GPRF:MEAS{instance}:FFTS:POW:CURR?", "Access"=0, "Range Table"="", "Read Callback"="", "Write Callback"="", "Supported Models"="", "Instrument Options"="", "Flags"=0, "Help"="Returns the traces of the spectrum diagram. The current, average, minimum and maximum traces can be retrieved.\nEach trace contains 801 power values and covers the configured frequency span.\n\nAvailable Repeated Capabilities:\ninstance: i0, i1, i2, i3, i4, i5, i6, i7, i8, i9, i10, i11, i12, i13, i14, i15, i16, i17, i18, i19, i20, i21, i22, i23, i24, i25, i26, i27, i28, i29, i30, i31, i32\r\n\nRemote-control command(s):\nREAD:GPRF:MEAS<i>:FFTSanalyzer:POWer:CURRent?"}, {"Level"=3, "Class Only"=FALSE, "Identifier"="RSCMXPGPRF_ATTR_READ_FFT_MEASUREMENT_POWER_AVERAGE", "Descriptive Name"="Read FFT Measurement Power Average", "Data Type"=6, "Command"="READ:GPRF:MEAS{instance}:FFTS:POW:AVER?", "Access"=0, "Range Table"="", "Read Callback"="", "Write Callback"="", "Supported Models"="", "Instrument Options"="", "Flags"=0, "Help"="Returns the traces of the spectrum diagram. The current, average, minimum and maximum traces can be retrieved.\nEach trace contains 801 power values and covers the configured frequency span.\n\nAvailable Repeated Capabilities:\ninstance: i0, i1, i2, i3, i4, i5, i6, i7, i8, i9, i10, i11, i12, i13, i14, i15, i16, i17, i18, i19, i20, i21, i22, i23, i24, i25, i26, i27, i28, i29, i30, i31, i32\r\n\nRemote-control command(s):\nREAD:GPRF:MEAS<i>:FFTSanalyzer:POWer:AVERage?"}, {"Level"=3, "Class Only"=FALSE, "Identifier"="RSCMXPGPRF_ATTR_READ_FFT_MEASUREMENT_POWER_MINIMUM", "Descriptive Name"="Read FFT Measurement Power Minimum", "Data Type"=6, "Command"="READ:GPRF:MEAS{instance}:FFTS:POW:MIN?", "Access"=0, "Range Table"="", "Read Callback"="", "Write Callback"="", "Supported Models"="", "Instrument Options"="", "Flags"=0, "Help"="Returns the traces of the spectrum diagram. The current, average, minimum and maximum traces can be retrieved.\nEach trace contains 801 power values and covers the configured frequency span.\n\nAvailable Repeated Capabilities:\ninstance: i0, i1, i2, i3, i4, i5, i6, i7, i8, i9, i10, i11, i12, i13, i14, i15, i16, i17, i18, i19, i20, i21, i22, i23, i24, i25, i26, i27, i28, i29, i30, i31, i32\r\n\nRemote-control command(s):\nREAD:GPRF:MEAS<i>:FFTSanalyzer:POWer:MINimum?"}, {"Level"=3, "Class Only"=FALSE, "Identifier"="RSCMXPGPRF_ATTR_READ_FFT_MEASUREMENT_POWER_MAXIMUM", "Descriptive Name"="Read FFT Measurement Power Maximum", "Data Type"=6, "Command"="READ:GPRF:MEAS{instance}:FFTS:POW:MAX?", "Access"=0, "Range Table"="", "Read Callback"="", "Write Callback"="", "Supported Models"="", "Instrument Options"="", "Flags"=0, "Help"="Returns the traces of the spectrum diagram. The current, average, minimum and maximum traces can be retrieved.\nEach trace contains 801 power values and covers the configured frequency span.\n\nAvailable Repeated Capabilities:\ninstance: i0, i1, i2, i3, i4, i5, i6, i7, i8, i9, i10, i11, i12, i13, i14, i15, i16, i17, i18, i19, i20, i21, i22, i23, i24, i25, i26, i27, i28, i29, i30, i31, i32\r\n\nRemote-control command(s):\nREAD:GPRF:MEAS<i>:FFTSanalyzer:POWer:MAXimum?"}, {"Level"=3, "Class Only"=FALSE, "Identifier"="RSCMXPGPRF_ATTR_FETCH_FFT_MEASUREMENT_POWER_CURRENT", "Descriptive Name"="Fetch FFT Measurement Power Current", "Data Type"=6, "Command"="FETC:GPRF:MEAS{instance}:FFTS:POW:CURR?", "Access"=0, "Range Table"="", "Read Callback"="", "Write Callback"="", "Supported Models"="", "Instrument Options"="", "Flags"=0, "Help"="Returns the traces of the spectrum diagram. The current, average, minimum and maximum traces can be retrieved.\nEach trace contains 801 power values and covers the configured frequency span.\n\nAvailable Repeated Capabilities:\ninstance: i0, i1, i2, i3, i4, i5, i6, i7, i8, i9, i10, i11, i12, i13, i14, i15, i16, i17, i18, i19, i20, i21, i22, i23, i24, i25, i26, i27, i28, i29, i30, i31, i32\r\n\nRemote-control command(s):\nFETCh:GPRF:MEAS<i>:FFTSanalyzer:POWer:CURRent?"}, {"Level"=3, "Class Only"=FALSE, "Identifier"="RSCMXPGPRF_ATTR_FETCH_FFT_MEASUREMENT_POWER_AVERAGE", "Descriptive Name"="Fetch FFT Measurement Power Average", "Data Type"=6, "Command"="FETC:GPRF:MEAS{instance}:FFTS:POW:AVER?", "Access"=0, "Range Table"="", "Read Callback"="", "Write Callback"="", "Supported Models"="", "Instrument Options"="", "Flags"=0, "Help"="Returns the traces of the spectrum diagram. The current, average, minimum and maximum traces can be retrieved.\nEach trace contains 801 power values and covers the configured frequency span.\n\nAvailable Repeated Capabilities:\ninstance: i0, i1, i2, i3, i4, i5, i6, i7, i8, i9, i10, i11, i12, i13, i14, i15, i16, i17, i18, i19, i20, i21, i22, i23, i24, i25, i26, i27, i28, i29, i30, i31, i32\r\n\nRemote-control command(s):\nFETCh:GPRF:MEAS<i>:FFTSanalyzer:POWer:AVERage?"}, {"Level"=3, "Class Only"=FALSE, "Identifier"="RSCMXPGPRF_ATTR_FETCH_FFT_MEASUREMENT_POWER_MINIMUM", "Descriptive Name"="Fetch FFT Measurement Power Minimum", "Data Type"=6, "Command"="FETC:GPRF:MEAS{instance}:FFTS:POW:MIN?", "Access"=0, "Range Table"="", "Read Callback"="", "Write 
